vi "Next Step.vi"(8 "error in (no error)":errorcluster, 11 "Actor in":refnum<class "Actor.lvclass">) -> (0 "error out":errorcluster, 2 "Next Step":string, 3 "Actor out":refnum<class "Actor.lvclass">)   [LabVIEW 2020, in "RTAF.lvlib" / "Actor.lvclass"]
uses:
  Actor.lvclass
  Actor.lvclass/Actor.ctl
  Sequencer/Sequencer.lvclass/Sequencer.ctl
  Sequencer/Sequencer.lvclass
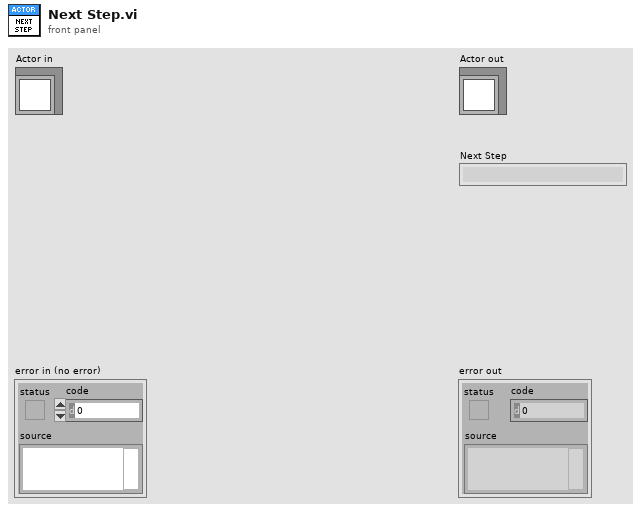
[diagram p1: front panel]
types:
  T1 = typedef "RTAF.lvlib/Sequencer.lvclass/Single Step Data.ctl" = cluster{"Name":string, "Parameter":variant, "Reply Channel":refnum<notifier>}
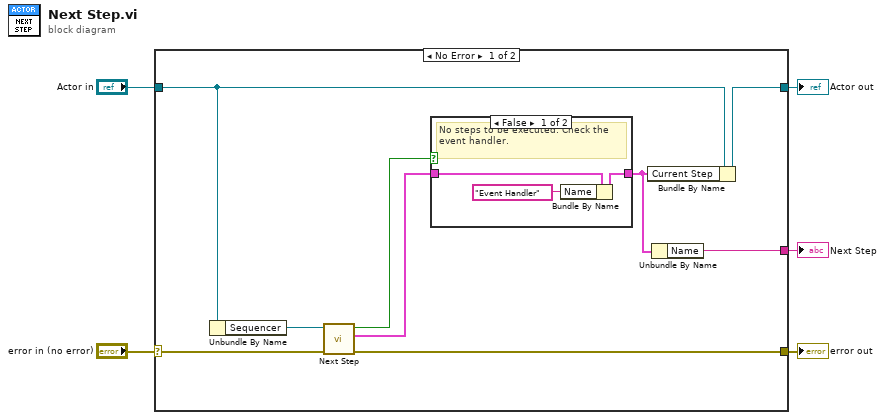
[diagram p0: block diagram]
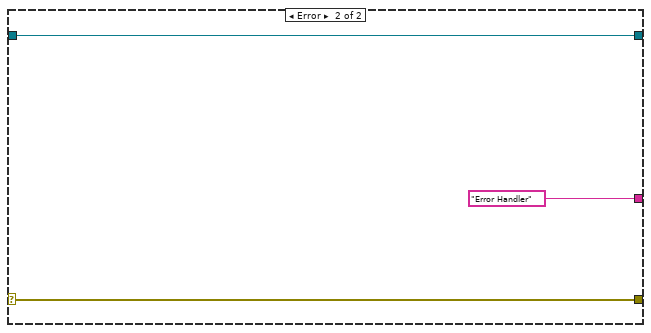
[diagram p3: hidden frame]
diagram:
  n1 = case shown="No Error" "error in (no error)" {
    selector: "error in (no error)" -> [w14 w21]
    tunnel: [w13 w21] -> w4
    tunnel: [w10 w20] -> w2
    tunnel: "Actor in" -> [w11 w20]
    tunnel: [w9 "Error Handler" ("Name")] -> w1
    frame No Error {
      n2 = Unbundle By Name(w11) -> ("Sequencer"=w12:refnum<class "Sequencer.lvclass">)
      n3 = call "Next Step.vi"("error in (no error)"=w14, "Sequencer in"=w12) -> ("error out"=w13:errorcluster, "Next Step"=w8:T1, "Step Available"=w7:bool)  [unwired: 7 in]
      n4 = case shown="False" w7 {
        tunnel: w8 -> [w17 w18]
        tunnel: [w15 w18] -> w6
        frame False {
          # "No steps to be executed. Check the event handler."
          n5 = Bundle By Name(cluster=w17, "Name"="Event Handler" ("String")) -> (w15:T1)
        }
        frame True {
          # "Something to be done."
        }
      }
      n6 = Bundle By Name(cluster=w11, "Current Step"=w6) -> (w10:refnum<class "Actor.lvclass">)
      n7 = Unbundle By Name(w6) -> ("Name"=w9:string)
    }
    frame Error {
    }
  }
  "error out" <- w4
  "Actor out" <- w2
  "Next Step" <- w1
